vi "ArearToIndex.vi"(5 "Input cluster":T1, 7 "Size interval":dbl=100.0 format="%#_13g", 8 "Number of Containers":i32=30, 9 "Initial size":dbl) -> (2 "Container number":i32, 3 "Output cluster":T1)   [LabVIEW 2024]
panel:
  out "Upper range":dbl[](array[numeric])
  out "Lower range":dbl[](array[numeric])
  out "In Range?":bool[](array[boolean])
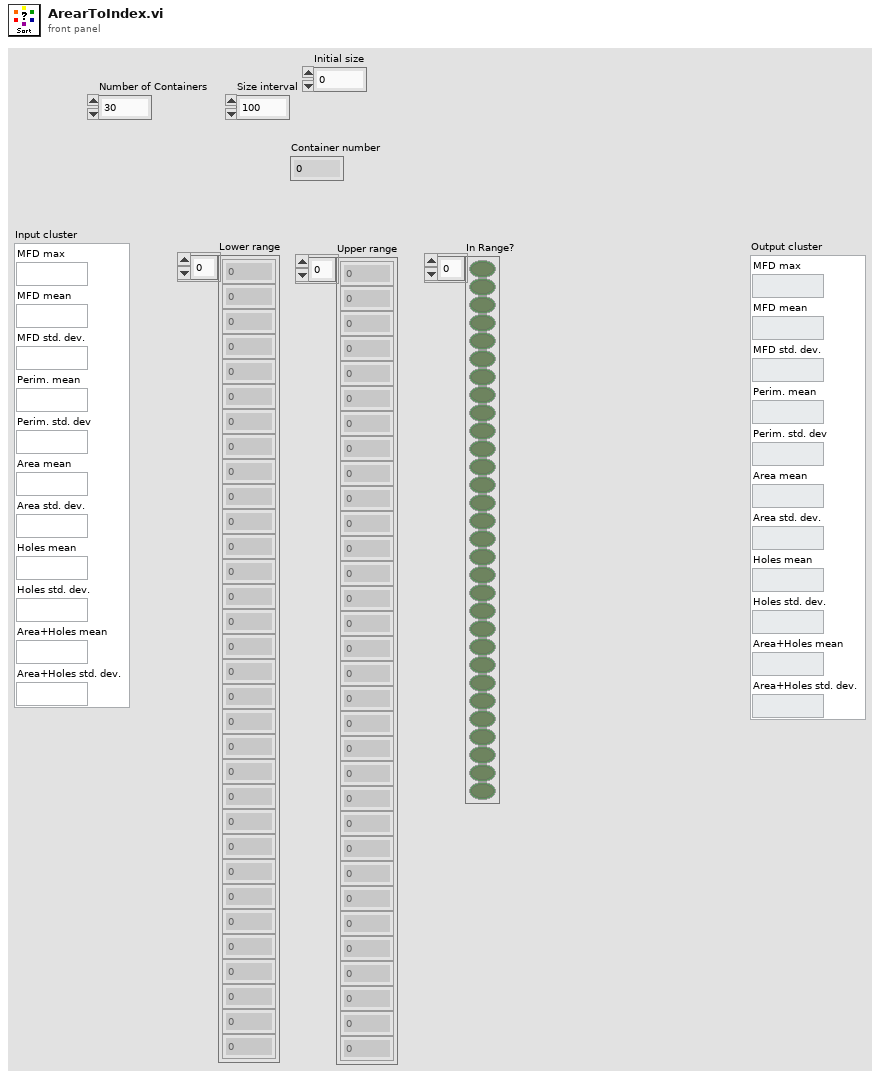
[diagram p1: front panel]
types:
  T1 = cluster{"MFD max":string, "MFD mean":string, "MFD std. dev.":string, "Perim. mean":string, "Perim. std. dev":string, "Area mean":string, "Area std. dev.":string, "Holes mean":string, "Holes std. dev.":string, "Area+Holes mean":string, "Area+Holes std. dev.":string}
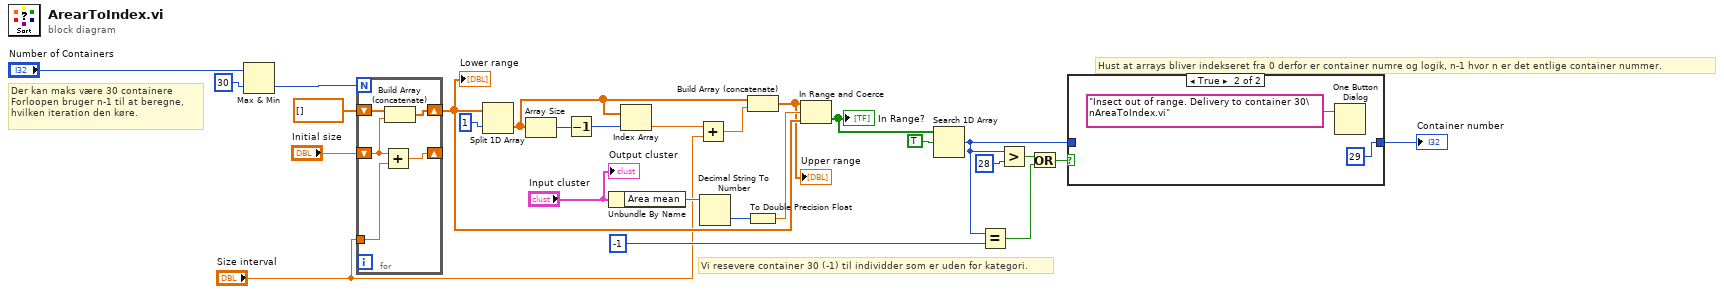
[diagram p0: block diagram]
diagram:
  # "Vi resevere container 30 (-1) til individder som er uden for kategori."
  # "Der kan maks være 30 containere\nForloopen bruger n-1 til at beregne, \nhvilken iteration den køre."
  # "Hust at arrays bliver indekseret fra 0 derfor er container numre og logik, n-1 hvor n er det entlige container nummer."
  n1 = Max & Min(x="Number of Containers", y=30) -> (min(x,y)=w10:i32)  [unwired: 1 out]
  n2 = for {
    N: w10 -> [_]
    shift-right: [w32] -> w8
    shift-left: dbl[] [] -> [w30]
    shift-right: [w31] -> _
    shift-left: "Initial size" -> [w29]
    tunnel: "Size interval" -> [w28]
    n3 = Add(x=w29, y=w28) -> (x+y=w31:dbl)
    n4 = Build Array (concatenate)(w30, w29) -> (w32:dbl[])
  }
  "Lower range" <- w8
  n5 = Split 1D Array(array=w8, index=1) -> (second subarray=w7:dbl[])  [unwired: 1 out]
  n6 = Array Size(array=w7) -> (size(s)=w3:i32)
  n7 = Decrement(x=w3) -> (x-1=w2:i32)
  n8 = Unbundle By Name("Input cluster") -> ("Area mean"=w22:string)
  n9 = Index Array(array=w7, index=w2) -> (element=w6:dbl)
  n10 = Add(x=w6, y="Size interval") -> (x+y=w4:dbl)
  n11 = Decimal String To Number(string=w22) -> (number=w21:i32)  [unwired: 2 in, 1 out]
  n12 = Build Array (concatenate)(w7, w4) -> (w1:dbl[])
  "Upper range" <- w1
  n13 = To Double Precision Float(number=w21) -> (double precision float=w20:dbl)
  n14 = In Range and Coerce(upper limit=w1, x=w20, lower limit=w8) -> (In Range?=w26:bool[])  [unwired: 1 out]
  "In Range?" <- w26
  n15 = Search 1D Array(1D array=w26, element=TRUE) -> (index of element=w13:i32)  [unwired: 1 in]
  n16 = Equal?(x=w13, y=-1) -> (x = y?=w14:bool)
  n17 = Greater?(x=w13, y=28) -> (0:w18:bool)
  n18 = Or(x=w18, y=w14) -> (x .or. y?=w15:bool)
  n19 = case shown="True" w15 {
    tunnel: w13 -> [w33 _]
    tunnel: [w33 29 ("index of element")] -> w12
    frame False {
    }
    frame True {
      n20 = One Button Dialog(message="Insect out of range. Delivery to container 30\nAreaToIndex.vi") -> ()  [unwired: 1 in, 1 out]
    }
  }
  "Container number" <- w12
  "Output cluster" <- "Input cluster"
